vi "delifbothzero.vi"(2 "in B":dbl[](array[numeric]), 3 "in A":dbl[](array[numeric])) -> (0 "out B":dbl[](array[numeric]), 1 "out A":dbl[](array[numeric]))   [LabVIEW 2017]
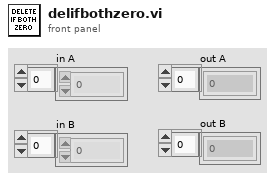
[diagram p1: front panel]
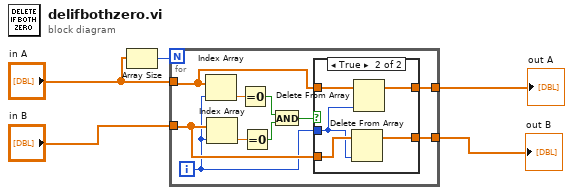
[diagram p0: block diagram]
diagram:
  n1 = Array Size(array="in A") -> (size(s)=w4:i32)
  n2 = for {
    N: w4 -> [_]
    tunnel: "in A" -> [w10]
    tunnel: "in B" -> [w9]
    tunnel: [w8] -> w3
    tunnel: [w7] -> w2
    i -> [w6]
    n3 = Index Array(array=w10, index=w6) -> (element=w15:dbl)
    n4 = Index Array(array=w9, index=w6) -> (element=w14:dbl)
    n5 = Equal To 0?(x=w15) -> (x = 0?=w12:bool)
    n6 = Equal To 0?(x=w14) -> (x = 0?=w13:bool)
    n7 = And(x=w12, y=w13) -> (x .and. y?=w11:bool)
    n8 = case shown="True" w11 {
      tunnel: w10 -> [w17 w21]
      tunnel: w9 -> [w16 w20]
      tunnel: [w17 w22] -> w8
      tunnel: [w16 w19] -> w7
      tunnel: w6 -> [_ w18]
      frame False {
      }
      frame True {
        n9 = Delete From Array(array=w20, index=w18) -> (array with subset deleted=w19:dbl[])  [unwired: 1 in, 1 out]
        n10 = Delete From Array(array=w21, index=w18) -> (array with subset deleted=w22:dbl[])  [unwired: 1 in, 1 out]
      }
    }
  }
  "out A" <- w3
  "out B" <- w2
